vi "8CHDAQ - Update Plot Ledgend and Scale.vi"(10 "Max":dbl, 11 "Channel Data":T1) -> ()   [LabVIEW 2015]
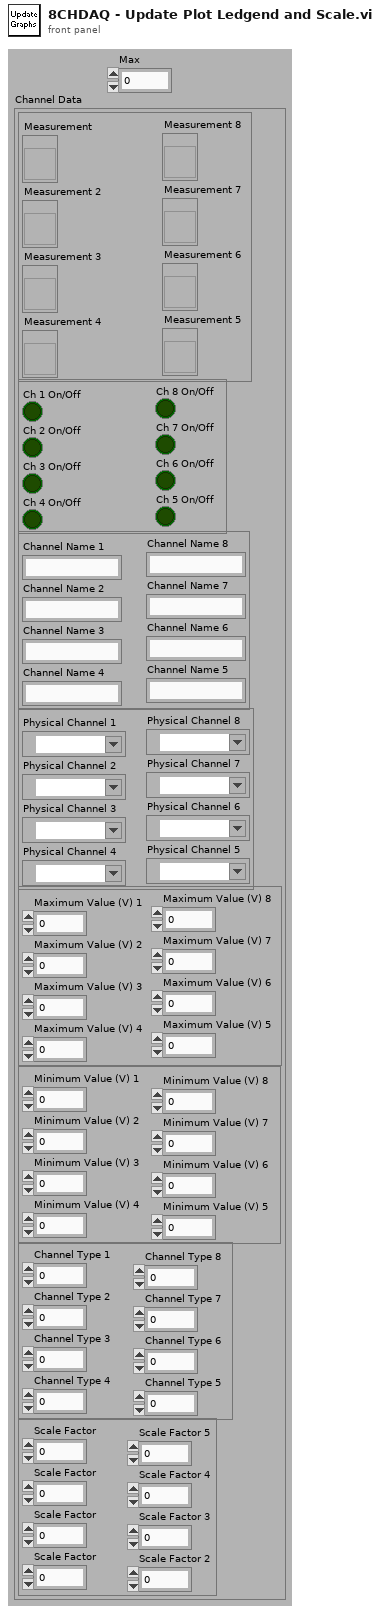
[diagram p1: front panel]
types:
  T1 = cluster{cluster{"Measurement":refnum<vi>, "Measurement 2":refnum<vi>, "Measurement 3":refnum<vi>, "Measurement 4":refnum<vi>, "Measurement 5":refnum<vi>, "Measurement 6":refnum<vi>, "Measurement 7":refnum<vi>, "Measurement 8":refnum<vi>}, cluster{"Ch 1 On/Off":bool, "Ch 2 On/Off":bool, "Ch 3 On/Off":bool, "Ch 4 On/Off":bool, "Ch 5 On/Off":bool, "Ch 6 On/Off":bool, "Ch 7 On/Off":bool, "Ch 8 On/Off":bool}, cluster{"Channel Name 1":string, "Channel Name 2":string, "Channel Name 3":string, "Channel Name 4":string, "Channel Name 5":string, "Channel Name 6":string, "Channel Name 7":string, "Channel Name 8":string}, cluster{"Physical Channel 1":tag, "Physical Channel 2":tag, "Physical Channel 3":tag, "Physical Channel 4":tag, "Physical Channel 5":tag, "Physical Channel 6":tag, "Physical Channel 7":tag, "Physical Channel 8":tag}, cluster{"Maximum Value (V) 1":dbl, "Maximum Value (V) 2":dbl, "Maximum Value (V) 3":dbl, "Maximum Value (V) 4":dbl, "Maximum Value (V) 5":dbl, "Maximum Value (V) 6":dbl, "Maximum Value (V) 7":dbl, "Maximum Value (V) 8":dbl}, cluster{"Minimum Value (V) 1":dbl, "Minimum Value (V) 2":dbl, "Minimum Value (V) 3":dbl, "Minimum Value (V) 4":dbl, "Minimum Value (V) 5":dbl, "Minimum Value (V) 6":dbl, "Minimum Value (V) 7":dbl, "Minimum Value (V) 8":dbl}, cluster{"Channel Type 1":u16, "Channel Type 2":u16, "Channel Type 3":u16, "Channel Type 4":u16, "Channel Type 5":u16, "Channel Type 6":u16, "Channel Type 7":u16, "Channel Type 8":u16}, cluster{"Scale Factor":dbl[unit], "Scale Factor":dbl[unit], "Scale Factor":dbl[unit], "Scale Factor":dbl[unit], "Scale Factor 2":dbl[unit], "Scale Factor 3":dbl[unit], "Scale Factor 4":dbl[unit], "Scale Factor 5":dbl[unit]}}
  T2 = cluster{"Measurement":refnum<vi>, "Measurement 2":refnum<vi>, "Measurement 3":refnum<vi>, "Measurement 4":refnum<vi>, "Measurement 5":refnum<vi>, "Measurement 6":refnum<vi>, "Measurement 7":refnum<vi>, "Measurement 8":refnum<vi>}
  T3 = cluster{"Ch 1 On/Off":bool, "Ch 2 On/Off":bool, "Ch 3 On/Off":bool, "Ch 4 On/Off":bool, "Ch 5 On/Off":bool, "Ch 6 On/Off":bool, "Ch 7 On/Off":bool, "Ch 8 On/Off":bool}
  T4 = cluster{"Channel Name 1":string, "Channel Name 2":string, "Channel Name 3":string, "Channel Name 4":string, "Channel Name 5":string, "Channel Name 6":string, "Channel Name 7":string, "Channel Name 8":string}
  T5 = cluster{"Channel Type 1":u16, "Channel Type 2":u16, "Channel Type 3":u16, "Channel Type 4":u16, "Channel Type 5":u16, "Channel Type 6":u16, "Channel Type 7":u16, "Channel Type 8":u16}
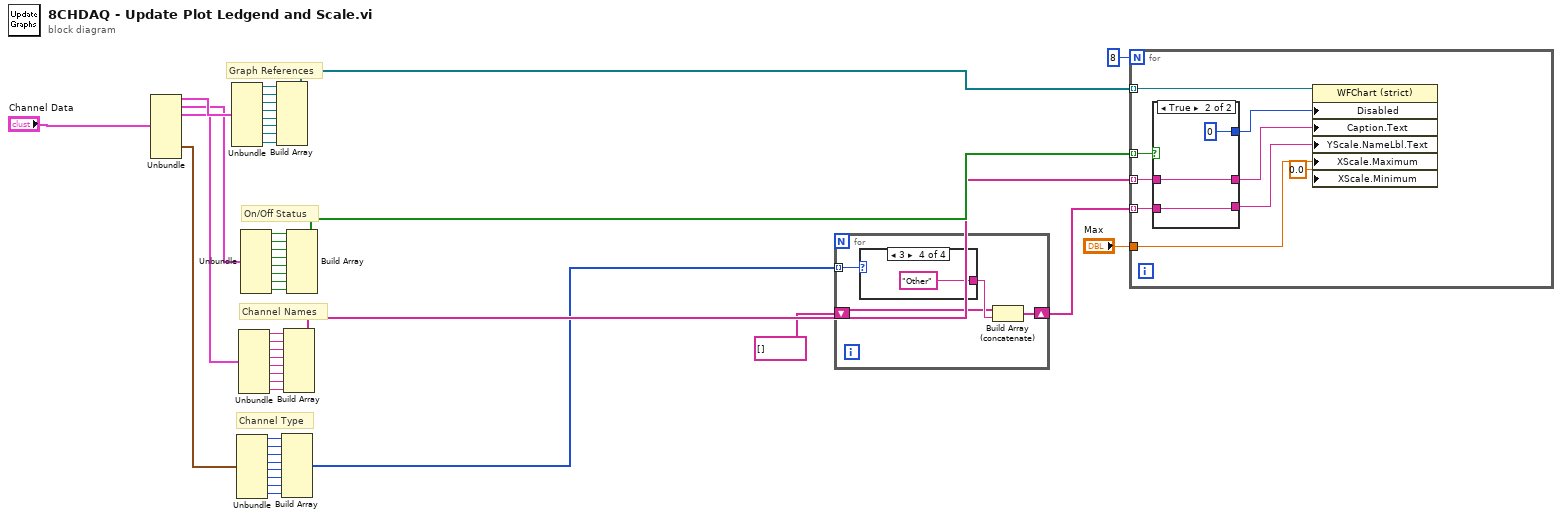
[diagram p0: block diagram]
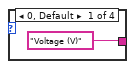
[diagram p2: hidden frame]
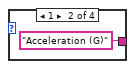
[diagram p3: hidden frame]
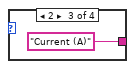
[diagram p4: hidden frame]
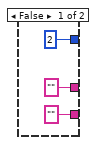
[diagram p5: hidden frame]
diagram:
  # "Channel Type"
  # "Channel Names"
  # "On/Off Status"
  # "Graph References"
  n1 = Unbundle("Channel Data") -> (w44:T2, w29:T3, w34:T4, w23:T5)  [unwired: 4 out]
  n2 = Unbundle(w44) -> ("Measurement"=w43:refnum<vi>, "Measurement 2"=w42:refnum<vi>, "Measurement 3"=w41:refnum<vi>, "Measurement 4"=w40:refnum<vi>, "Measurement 5"=w4:refnum<vi>, "Measurement 6"=w3:refnum<vi>, "Measurement 7"=w2:refnum<vi>, "Measurement 8"=w1:refnum<vi>)
  n3 = Unbundle(w23) -> ("Channel Type 1"=w22:u16, "Channel Type 2"=w26:u16, "Channel Type 3"=w25:u16, "Channel Type 4"=w24:u16, "Channel Type 5"=w16:u16, "Channel Type 6"=w15:u16, "Channel Type 7"=w14:u16, "Channel Type 8"=w13:u16)
  n4 = Unbundle(w34) -> ("Channel Name 1"=w35:string, "Channel Name 2"=w36:string, "Channel Name 3"=w37:string, "Channel Name 4"=w38:string, "Channel Name 5"=w12:string, "Channel Name 6"=w11:string, "Channel Name 7"=w10:string, "Channel Name 8"=w9:string)
  n5 = Unbundle(w29) -> ("Ch 1 On/Off"=w30:bool, "Ch 2 On/Off"=w31:bool, "Ch 3 On/Off"=w32:bool, "Ch 4 On/Off"=w33:bool, "Ch 5 On/Off"=w8:bool, "Ch 6 On/Off"=w7:bool, "Ch 7 On/Off"=w6:bool, "Ch 8 On/Off"=w5:bool)
  n6 = Build Array(w43, w42, w41, w40, w4, w3, w2, w1) -> (w39:refnum<vi>[])
  n7 = Build Array(w22, w26, w25, w24, w16, w15, w14, w13) -> (w21:u16[])
  n8 = Build Array(w35, w36, w37, w38, w12, w11, w10, w9) -> (w27:string[])
  n9 = Build Array(w30, w31, w32, w33, w8, w7, w6, w5) -> (w28:bool[])
  n10 = for {
    tunnel: w21 -> [w49] mode=indexing
    shift-right: [w48] -> w19
    shift-left: string[] [] -> [w46]
    n11 = case shown="3" w49 {
      tunnel: ["Voltage (V)" "Acceleration (G)" "Current (A)" "Other"] -> w47
      frame 0, Default {
      }
      frame 1 {
      }
      frame 2 {
      }
      frame 3 {
      }
    }
    n12 = Build Array (concatenate)(w46, w47) -> (w48:string[])
  }
  n13 = for {
    N: 8 -> [_]
    tunnel: w39 -> [w62] mode=indexing
    tunnel: w28 -> [w58] mode=indexing
    tunnel: w27 -> [w57] mode=indexing
    tunnel: w19 -> [w56] mode=indexing
    tunnel: "Max" -> [w55]
    n14 = case shown="True" w58 {
      tunnel: [2 0] -> w61
      tunnel: ["" w66] -> w60
      tunnel: ["" w67] -> w59
      tunnel: w56 -> [_ w67]
      tunnel: w57 -> [_ w66]
      frame False {
      }
      frame True {
      }
    }
    n15 = property on="Property Node" class="WFChart (strict)"(reference=w62, "Disabled"=w61, "Caption.Text"=w60, "YScale.NameLbl.Text"=w59, "XScale.Maximum"=w55, "XScale.Minimum"=0.0 ("X Scale.Range:Minimum")) -> ()  [unwired: 1 in, 2 out]
  }
